vi "Current Limit.vi"(0 "Current Limit Parameters":T3 {"Min Cell Voltage Actual Value" format="%#.2f"; "Max Cell Voltage Actual Value" format="%#.2f"}, 1 "Current Limit":dbl=83.0 format="%#_13g", 5 "Current In":dbl, 7 "Real Time State":T1, 11 "Error In":errorcluster) -> (4 "Limited?":bool=TRUE, 8 "Current Out":dbl, 10 "Current Limit Output":T2, 15 "Error Out":errorcluster)   [LabVIEW 2014]
uses:
  Controls/Current Limit Parameters.ctl
  Controls/Current Limit Output.ctl
  Controls/RT State.ctl
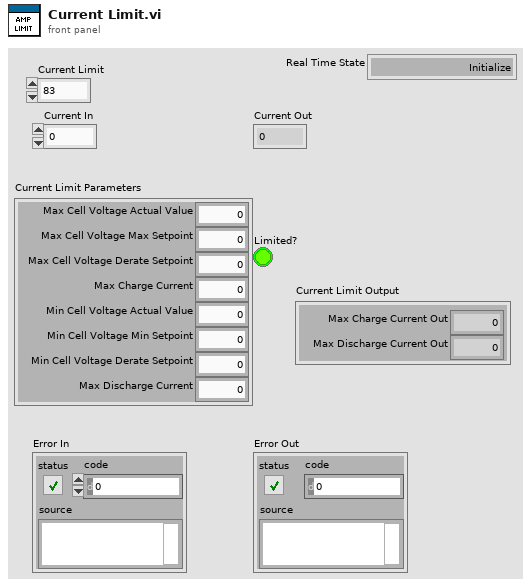
[diagram p1: front panel]
types:
  T1 = typedef "RT State.ctl" = enum16{"Initialize", "Ready", "Startup 1 - Start Genset", "Startup 2 - Start Inverter", "Startup 3 - Battery Match", "SpotGen - Start", "SpotGen - Charge", "SpotGen - Desync", "SpotGen - Discharge", "SpotGen - Sync", "Shutdown", "INVALID STATE"}
  T2 = typedef "Current Limit Output.ctl" = cluster{"Max Charge Current Out":dbl, "Max Discharge Current Out":dbl}
  T3 = typedef "Current Limit Parameters.ctl" = cluster{"Max Cell Voltage Max Setpoint":dbl, "Max Cell Voltage Actual Value":dbl, "Max Cell Voltage Derate Setpoint":dbl, "Max Charge Current":dbl, "Min Cell Voltage Min Setpoint":dbl, "Min Cell Voltage Actual Value":dbl, "Min Cell Voltage Derate Setpoint":dbl, "Max Discharge Current":dbl}
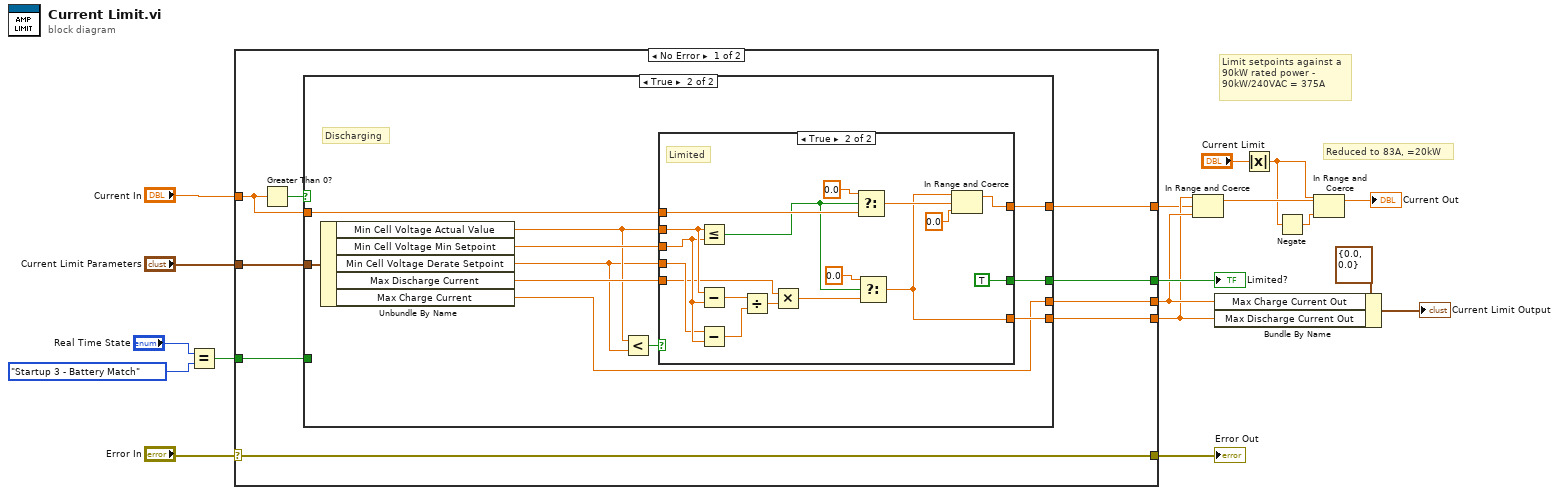
[diagram p0: block diagram]
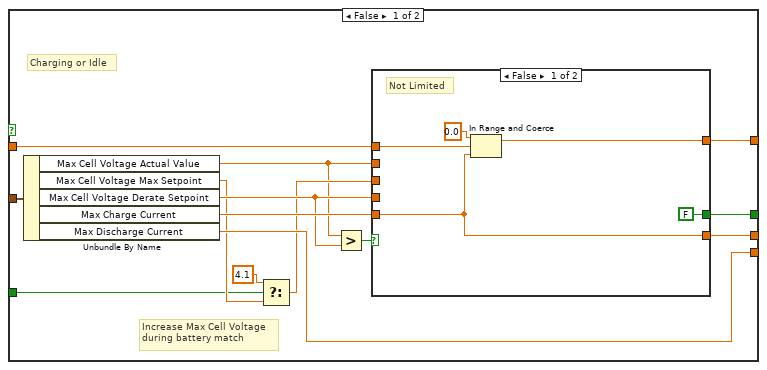
[diagram p2: hidden frame]
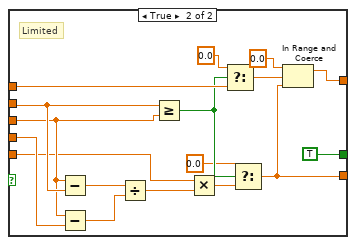
[diagram p3: hidden frame]
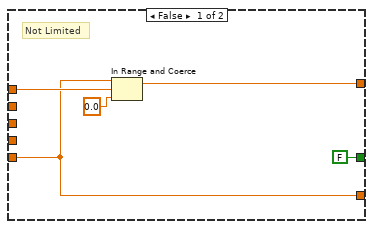
[diagram p4: hidden frame]
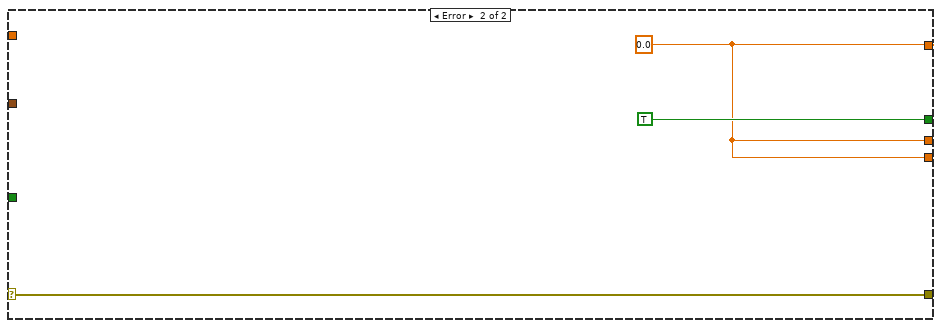
[diagram p5: hidden frame]
diagram:
  # "Reduced to 83A, =20kW"
  # "Limit setpoints against a\n90kW rated power -\n90kW/240VAC = 375A"
  n1 = Equal?(x="Real Time State", y=RT_State."Startup 3 - Battery Match") -> (x = y?=w4:bool)
  n2 = case shown="No Error" "Error In" {
    selector: "Error In" -> [w26 w99]
    tunnel: [w22 w97] -> w9
    tunnel: "Current In" -> [w27 _]
    tunnel: [w26 w99] -> w16
    tunnel: [w25 TRUE] -> w15
    tunnel: "Current Limit Parameters" -> [w24 _]
    tunnel: [w23 w97] -> w11
    tunnel: [w21 w97] -> w10
    tunnel: w4 -> [w19 _]
    frame No Error {
      n3 = Greater Than 0?(x=w27) -> (x > 0?=w20:bool)
      n4 = case shown="True" w20 {
        tunnel: w27 -> [w41 w64]
        tunnel: [w39 w73] -> w22
        tunnel: [w38 w72] -> w25
        tunnel: w24 -> [w37 w71]
        tunnel: [w34 w65] -> w23
        tunnel: [w33 w66] -> w21
        tunnel: w19 -> [w29 _]
        frame False {
          # "Increase Max Cell Voltage\nduring battery match"
          # "Charging or Idle"
          n5 = Unbundle By Name(w37) -> ("Max Cell Voltage Actual Value"=w28:dbl, "Max Cell Voltage Max Setpoint"=w31:dbl, "Max Cell Voltage Derate Setpoint"=w35:dbl, "Max Charge Current"=w36:dbl, "Max Discharge Current"=w33:dbl)
          n6 = Select(t=4.1, s=w29, f=w31) -> (s? t:f=w30:dbl)
          n7 = Greater?(x=w28, y=w35) -> (0:w40:bool)
          n8 = case shown="False" w40 {
            tunnel: w41 -> [w45 w57]
            tunnel: [w43 w60] -> w39
            tunnel: [FALSE TRUE] -> w38
            tunnel: w36 -> [w42 w51]
            tunnel: w28 -> [_ w54]
            tunnel: w30 -> [_ w53]
            tunnel: w35 -> [_ w52]
            tunnel: [w42 w47] -> w34
            frame False {
              # "Not Limited"
              n9 = In Range and Coerce(upper limit=0.0, x=w45, lower limit=w42) -> (coerced(x)=w43:dbl)  [unwired: 1 out]
            }
            frame True {
              # "Limited"
              n10 = Subtract(x=w53, y=w54) -> (x-y=w63:dbl)
              n11 = Subtract(x=w53, y=w52) -> (x-y=w62:dbl)
              n12 = Divide(x=w63, y=w62) -> (x/y=w61:dbl)
              n13 = Greater Or Equal?(x=w54, y=w53) -> (x >= y?=w50:bool)
              n14 = Multiply(x=w51, y=w61) -> (x*y=w48:dbl)
              n15 = Select(t=0.0, s=w50, f=w57) -> (s? t:f=w59:dbl)
              n16 = Select(t=0.0, s=w50, f=w48) -> (s? t:f=w47:dbl)
              n17 = In Range and Coerce(upper limit=0.0 ("lower limit"), x=w59, lower limit=w47) -> (coerced(x)=w60:dbl)  [unwired: 1 out]
            }
          }
        }
        frame True {
          # "Discharging"
          n18 = Unbundle By Name(w71) -> ("Min Cell Voltage Actual Value"=w68:dbl, "Min Cell Voltage Min Setpoint"=w70:dbl, "Min Cell Voltage Derate Setpoint"=w67:dbl, "Max Discharge Current"=w69:dbl, "Max Charge Current"=w65:dbl)
          n19 = Less?(x=w68, y=w67) -> (x < y?=w74:bool)
          n20 = case shown="True" w74 {
            tunnel: w64 -> [w78 w90]
            tunnel: [w77 w92] -> w73
            tunnel: [FALSE TRUE] -> w72
            tunnel: w68 -> [_ w87]
            tunnel: w70 -> [_ w86]
            tunnel: w67 -> [_ w85]
            tunnel: w69 -> [w75 w84]
            tunnel: [w75 w80] -> w66
            frame False {
              # "Not Limited"
              n21 = In Range and Coerce(upper limit=w75, x=w78, lower limit=0.0) -> (coerced(x)=w77:dbl)  [unwired: 1 out]
            }
            frame True {
              # "Limited"
              n22 = Less Or Equal?(x=w87, y=w86) -> (x <= y?=w82:bool)
              n23 = Subtract(x=w87, y=w86) -> (x-y=w96:dbl)
              n24 = Subtract(x=w85, y=w86) -> (x-y=w95:dbl)
              n25 = Divide(x=w96, y=w95) -> (x/y=w94:dbl)
              n26 = Multiply(x=w84, y=w94) -> (x*y=w81:dbl)
              n27 = Select(t=0.0, s=w82, f=w90) -> (s? t:f=w91:dbl)
              n28 = Select(t=0.0, s=w82, f=w81) -> (s? t:f=w80:dbl)
              n29 = In Range and Coerce(upper limit=w80, x=w91, lower limit=0.0 ("upper limit")) -> (coerced(x)=w92:dbl)  [unwired: 1 out]
            }
          }
        }
      }
    }
    frame Error {
      w97 = 0.0 ("t")
    }
  }
  "Error Out" <- w16
  "Limited?" <- w15
  n30 = In Range and Coerce(upper limit=w10, x=w9, lower limit=w11) -> (coerced(x)=w7:dbl)  [unwired: 1 out]
  n31 = Bundle By Name(cluster=T2 {"Max Charge Current Out"=0.0, "Max Discharge Current Out"=0.0} ("Current Limit Output"), "Max Charge Current Out"=w11, "Max Discharge Current Out"=w10) -> (→"Current Limit Output":T2)
  n32 = Absolute Value(x="Current Limit") -> (abs(x)=w2:dbl)
  n33 = Negate(x=w2) -> (-x=w3:dbl)
  n34 = In Range and Coerce(upper limit=w2, x=w7, lower limit=w3) -> (coerced(x)=→"Current Out":dbl)  [unwired: 1 out]
